vi "20211015_HW00.vi"() -> ()   [LabVIEW 2019]
panel:
  out "Time":timestamp format="%<%x %.3X>T"
  out "Clock":T1(knob)={"Numeric"=0.0, "Numeric"=0.0, "Numeric"=6.0} scale=0.0..12.0
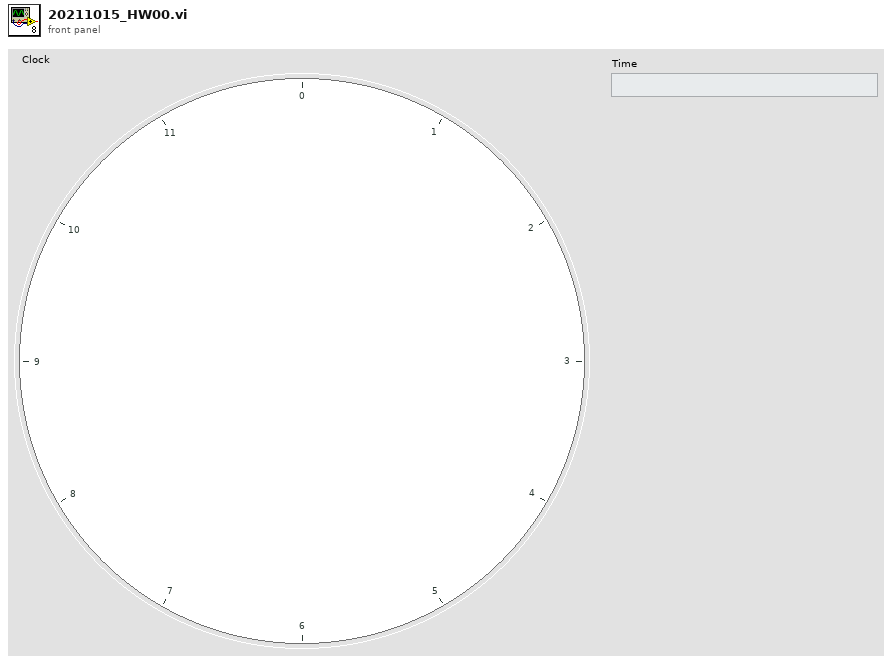
[diagram p1: front panel]
types:
  T1 = cluster{"Numeric":dbl, "Numeric":dbl, "Numeric":dbl}
  T2 = typedef "LVDateTimeRec.ctl" = cluster{"fractional second":dbl, "second":i32, "minute":i32, "hour":i32, "day of month":i32, "month":i32, "year":i32, "day of week":i32, "day of year":i32, "DST":i32}
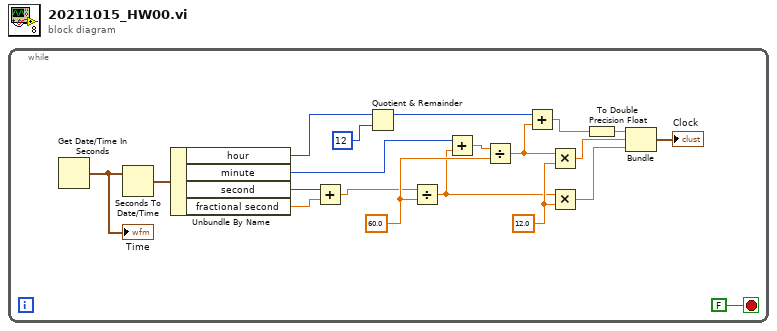
[diagram p0: block diagram]
diagram:
  n1 = while {
    stop <- FALSE stop-if-true
    w17 = 12.0 ("y")
    w18 = 60.0 ("y")
    n2 = Get Date/Time In Seconds() -> (seconds since 1Jan1904=w13:timestamp)
    "Time" <- w13
    n3 = Seconds To Date/Time(time stamp (now)=w13) -> (date time rec=w20:T2)  [unwired: 1 in]
    n4 = Unbundle By Name(w20) -> ("hour"=w10:i32, "minute"=w7:i32, "second"=w8:i32, "fractional second"=w12:dbl)
    n5 = Add(x=w8, y=w12) -> (x+y=w11:dbl)
    n6 = Quotient & Remainder(x=w10, y=12) -> (x-y*floor(x/y)=w5:i32)  [unwired: 1 out]
    n7 = Divide(x=w11, y=w18) -> (x/y=w6:dbl)
    n8 = Add(x=w7, y=w6) -> (x+y=w4:dbl)
    n9 = Divide(x=w4, y=w18) -> (x/y=w2:dbl)
    n10 = Add(x=w5, y=w2) -> (x+y=w3:dbl)
    n11 = Multiply(x=w2, y=w17) -> (x*y=w16:dbl)
    n12 = Multiply(x=w6, y=w17) -> (x*y=w15:dbl)
    n13 = To Double Precision Float(number=w3) -> (double precision float=w14:dbl)
    n14 = Bundle(w14, w16, w15) -> (→"Clock":cluster{dbl, dbl, dbl})  [unwired: 1 in]
  }
